vi "Meas Gen Path.vi"(8 "f id":i32, 9 "n id":i32, 11 "swp cfg":T1 {"f list"."bias" format="%#_3p"; "f list"."level" format="%#_3p"; "f list"."fs [Hz]" format="%#_5p"; "f list"."time [s]" format="%#_3p"; "f list"."f/fs" format="%#_3p"; "f list"."periods" format="%#_3f"; "f list"."f [Hz]" format="%#_5p"}) -> (3 "meas path":path)   [LabVIEW 2013]
doc: "Generate measurement path from sweep setup and sweep spot indices."
uses:
  Meas Sweep Config.ctl
  Meas Freq Info.ctl
  meas_swp_mode.ctl
  meas_sweep_flist_mode.ctl
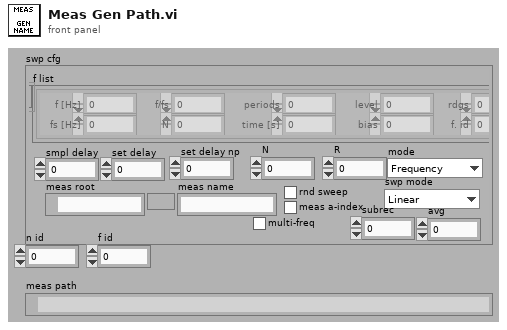
[diagram p1: front panel]
types:
  T1 = typedef "Meas Sweep Config.ctl" = cluster{"N":i32, "R":i32, "f list":T2[], "smpl delay":dbl, "set delay":dbl, "set delay np":dbl, "meas root":path, "meas name":string, "meas a-index":bool, "rnd sweep":bool, "mode":T3, "swp mode":T4, "avg":i32, "subrec":i32, "multi-freq":bool}
  T2 = typedef "Meas Freq Info.ctl" = cluster{"f [Hz]":dbl, "periods":dbl, "f/fs":dbl, "time [s]":dbl, "fs [Hz]":dbl, "N":i32, "level":dbl, "bias":dbl, "rdgs":i32, "f. id":i32}
  T3 = typedef "meas_swp_mode.ctl" = enum16{"Frequency", "Level", "Bias"}
  T4 = typedef "meas_sweep_flist_mode.ctl" = enum16{"Linear", "Log10"}
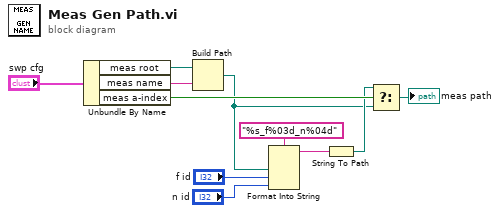
[diagram p0: block diagram]
diagram:
  n1 = Unbundle By Name("swp cfg") -> ("meas root"=w10:path, "meas name"=w9:string, "meas a-index"=w5:bool)
  n2 = Build Path(base path=w10, name or relative path=w9) -> (appended path=w2:path)
  n3 = Format Into String(format string="%s_f%03d_n%04d", w2, "f id", "n id") -> (resulting string=w4:string)  [unwired: 2 in, 1 out]
  n4 = String To Path(string=w4) -> (path=w3:path)
  n5 = Select(t=w3, s=w5, f=w2) -> (s? t:f=→"meas path":path)
